vi "Check.vi"() -> ()   [LabVIEW 2019]
uses:
  Y_SP.xctl
  Y_source.ctl
  95228b63-dbad-4f81-a48d-2b4403cca3b5.vi
  Heating.lvlib
panel:
  out "Numeric 3":dbl
  out "Numeric 2":dbl
  out "Numeric":dbl
  in  "SP":dbl
  in  "SP_Set":dbl
  in  "SP_Source":T1
  in  "connect":bool
  in  "Y_control":cluster{dbl, dbl, dbl}(xcontrol)
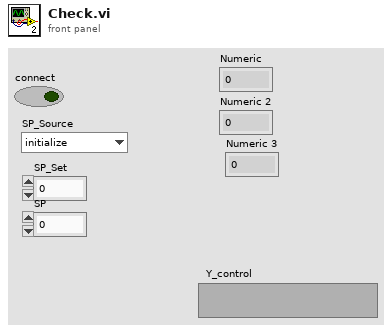
[diagram p1: front panel]
types:
  T1 = typedef "Heating.lvlib/Y_source.ctl" = enum8{"initialize", "local disabled", "local hand", "hand", "auto", "dist"}
  T2 = cluster{"connect":bool, "SP_Source":T1, "SP_Set":dbl, "SP":dbl}
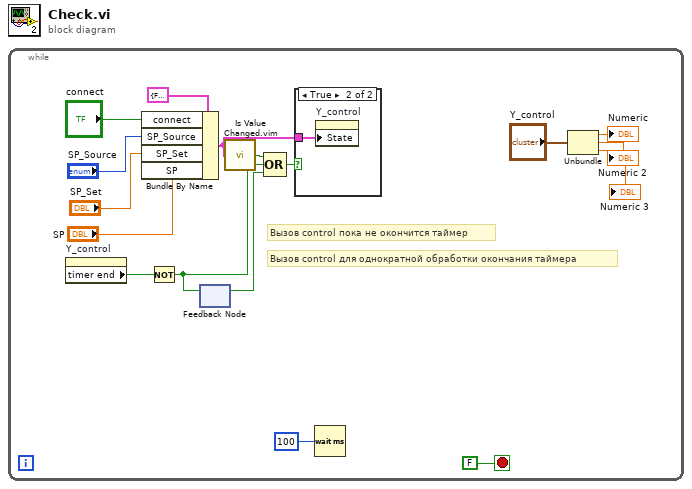
[diagram p0: block diagram]
diagram:
  n1 = while {
    stop <- FALSE stop-if-true
    # "Вызов control пока не окончится таймер"
    # "Вызов control для однократной обработки окончания таймера"
    n2 = property on="Y_control" class="Y_SP (strict)"() -> ("timer end"=w14:bool)  [unwired: 2 in, 2 out]
    n3 = Bundle By Name(cluster=T2 {"connect"=FALSE, "SP_Source"=enum."initialize", "SP_Set"=0.0, "SP"=0.0} ("source"), "connect"="connect", "SP_Source"="SP_Source", "SP_Set"="SP_Set", "SP"="SP") -> (w10:T2)
    n4 = Not(x=w14) -> (.not. x?=w12:bool)
    n5 = feedback-in #1(w12) -> ()
    n6 = feedback #1() -> (w13:bool)  [unwired: 1 in]
    n7 = call "Is Value Changed.vim"("value"=w10) -> ("changed or first call?"=w9:bool)
    n8 = Compound Arithmetic op=OR(w9, w12, w13) -> (w15:bool)
    n9 = case shown="True" w15 {
      tunnel: w10 -> [_ w18]
      frame False {
      }
      frame True {
        n10 = property on="Y_control" class="Y_SP (strict)"("State"=w18) -> ()  [unwired: 2 in, 2 out]
      }
    }
    n11 = Wait (ms)(milliseconds to wait=u32 100) -> ()  [unwired: 1 out]
    n12 = Unbundle("Y_control") -> (→"Numeric":dbl, →"Numeric 2":dbl, →"Numeric 3":dbl)
  }
